vi "APC_9049_SensorCalibration.vi"() -> (0 "DAQqueues":T1={"SignalList"={"CAS"=["Pcyl1_bar", "Pcyl2_bar", "Pcyl3_bar", "Pcyl4_bar", "Pcyl5_bar", "Pcyl6_bar", "Ppre_bar", "Psyst_bar", "Pexh_bar"], "CycAvg"=["TimeStamp9049_ms", "TimeStamp9056echo_ms", "InjectionState_b", "InjEnable_b", "MainEnable_b", "MainDuration_ms", "MainSOI_CADBTDC", "SparkEnable_b", "SparkTiming_CADBTDC", "EngineSpeed_rpm", "WF_PT_012avg_bar", "WF_PT_005avg_bar", "PrechamberPeakPdiff_bar", "IMEPg1_bar", "IMEPg2_bar", "IMEPg3_bar", "IMEPg4_bar", "IMEPg5_bar", "IMEPg6_bar", "IMEPn1_bar", "IMEPn2_bar", "IMEPn3_bar", "IMEPn4_bar", "IMEPn5_bar", "IMEPn6_bar", "PMEP1_bar", "PMEP2_bar", "PMEP3_bar", "PMEP4_bar", "PMEP5_bar", "PMEP6_bar", "MaxPcyl1_bar", "MaxPcyl2_bar", "MaxPcyl3_bar", "MaxPcyl4_bar", "MaxPcyl5_bar", "MaxPcyl6_bar", "IMEPstd1_bar", "IMEPstd2_bar", "IMEPstd3_bar", "IMEPstd4_bar", "IMEPstd5_bar", "IMEPstd6_bar", "MAPO1_bar", "MAPO2_bar", "MAPO3_bar", "MAPO4_bar", "MAPO5_bar", "MAPO6_bar", "RI1", "RI2", "RI3", "RI4", "RI5", "RI6", "maxQ1_J", "maxQ2_J", "maxQ3_J", "maxQ4_J", "maxQ5_J", "maxQ6_J", "CA03_1_CADATDC", "CA03_2_CADATDC", "CA03_3_CADATDC", "CA03_4_CADATDC", "CA03_5_CADATDC", "CA03_6_CADATDC", "CA10_1_CADATDC", "CA10_2_CADATDC", "CA10_3_CADATDC", "CA10_4_CADATDC", "CA10_5_CADATDC", "CA10_6_CADATDC", "CA50_1_CADATDC", "CA50_2_CADATDC", "CA50_3_CADATDC", "CA50_4_CADATDC", "CA50_5_CADATDC", "CA50_6_CADATDC", "CA90_1_CADATDC", "CA90_2_CADATDC", "CA90_3_CADATDC", "CA90_4_CADATDC", "CA90_5_CADATDC", "CA90_6_CADATDC", "CA97_1_CADATDC", "CA97_2_CADATDC", "CA97_3_CADATDC", "CA97_4_CADATDC", "CA97_5_CADATDC", "CA97_6_CADATDC", "CA10CA90_1_CAD", "CA10CA90_2_CAD", "CA10CA90_3_CAD", "CA10CA90_4_CAD", "CA10CA90_5_CAD", "CA10CA90_6_CAD", "maxdpdcad1_barCAD", "maxdpdcad2_barCAD", "maxdpdcad3_barCAD", "maxdpdcad4_barCAD", "maxdpdcad5_barCAD", "maxdpdcad6_barCAD", "kappa_comp1_r", "kappa_comp2_r", "kappa_comp3_r", "kappa_comp4_r", "kappa_comp5_r", "kappa_comp6_r", "kappa_exp1_r", "kappa_exp2_r", "kappa_exp3_r", "kappa_exp4_r", "kappa_exp5_r", "kappa_exp6_r", "CylPresWarnings_u64", "CylPresErrors_u64", "TimeStamp9056_ms", "SystemState_i8", "WF_PT_001_bar", "WF_OA_001_O2_perc", "WF_OA_001_O2corr_perc", "WF_OA_001_Lambda_r", "WF_OA_002_O2_perc", "WF_OA_002_Lambda_r", "WF_OA_002_NOx_ppm", "EO_PT_001_bar", "TORQUE_Nm", "NI9205_9_V", "NI9205_10_V", "NI9205_11_V", "NI9205_12_V", "NI9205_13_V", "NI9205_14_V", "NI9205_15_V", "NG_FT_001_kgs", "NG_PT_001_bar", "NGDI_PT_001_bar", "O2_FC_001_kgs", "NG_FC_001_kgs", "NGDI_FT_001_kgs", "WF_PT_004_bar", "O2_PT_001_bar", "AR_PT_001_bar", "AR_FT_001_kgs", "WF_PT_016_bar", "WF_PT_014_bar", "SW_FT_001_kgs", "SW_FT_002_kgs", "SW_FT_003_kgs", "SW_FT_004_kgs", "WF_TT_001_degC", "O2_TT_001_degC", "AR_TT_001_degC", "NG_TT_001_degC", "NGDI_TT_001_degC", "WF_TT_002 _degC", "WF_TT_003_degC", "WF_TT_004_degC", "WF_TT_007_degC", "PC_TT_001_degC", "PC_TT_002_degC", "PC_TT_003_degC", "PC_TT_004_degC", "PC_TT_005_degC", "PC_TT_006_degC", "EC_TT_001_degC", "EC_TT_002_degC", "SW_TT_001_degC", "SW_TT_002_degC", "SW_TT_003_degC", "SW_TT_004_degC", "SW_TT_005_degC", "SW_TT_006_degC", "SW_TT_007_degC", "SW_TT_008_degC", "SW_TT_009_degC", "EO_TT_001_degC", "EO_TT_002_degC", "NI9214b_13_degC", "NI9214b_14_degC", "NI9214b_15_degC", "NI9214b_16_degC", "NI9264_AO0_V", "NI9264_AO1_V", "NI9264_AO2_V", "NI9264_AO3_V", "NI9264_AO4_V", "NI9264_AO5_V", "NI9264_AO6_V", "NI9264_AO7_V", "NI9264_AO8_V", "NI9264_AO9_V", "NI9264_AO10_V", "NI9264_AO11_V", "NI9264_AO12_V", "NI9264_AO13_V", "NI9264_AO14_V", "NI9264_AO15_V", "O2_FC_001_REF_mA", "AR_PC_002_REF_mA", "NG_FC_001_REF_mA", "EC_FC_001_mA", "SW_FC_004_REF_mA", "SW_FC_009_mA", "DYNO_REF_mA", "NI9266_AO7_mA", "NG_FV_001_b", "O2_PV_004_b", "AR_PV_004_b", "WF_FC_001_b", "WF_FC_002_b", "WF_FC_003_b", "NI9375_AO6_b", "NI9375_AO7_b", "NI9375_AO8_b", "NI9375_AO9_b", "NI9375_AO10_b", "NI9375_AO11_b", "NI9375_AO12_b", "NI9375_AO13_b", "NI9375_AO14_b", "NI9375_AO15_b", "NI9375_AI0_b", "NI9375_AI1_b", "NI9375_AI2_b", "NI9375_AI3_b", "NI9375_AI4_b", "NI9375_AI5_b", "NI9375_AI6_b", "NI9375_AI7_b", "NI9375_AI8_b", "NI9375_AI9_b", "NI9375_AI10_b", "NI9375_AI11_b", "NI9375_AI12_b", "NI9375_AI13_b", "NI9375_AI14_b", "NI9375_AI15_b", "AIC103_CO2_ConcTarget_ack", "AT103_CO2Conc", "PV103_PressTarget_kPa_ack", "PT103_Pressure_kPa", "PV103_VlvPosTarget_pc_ack", "PV103_VlvPos_pc_fb", "AIC201_CO2_ConcTarget_ack", "AT201_CO2Conc", "FV301_FlowTarget_kgh_ack", "FT301_Flow_kgh", "FV301_VlvPosTarget_pc_ack", "FV301_VlvPos_pc_fb", "PV300_PressTarget_kPa_ack", "PT300_Pressure_kPa", "PV300_VlvPosTarget_pc_ack", "PV300_VlvPos_pc_fb", "C101_CompSpeed_rpm", "PT104_Pressure_kPa", "PT106_Pressure_kPa", "PLC_Manual_Control", "MTR_State", "MTR_HeartBeat", "PV103_Ctrl_Mode_act", "FV301_Ctrl_Mode_act", "PV300_Ctrl_Mode_act", "MTR_Diagnostic_Status"]}, "Queues"={"CAS"=refnum, "CycAvg"=refnum}, "scaled units"=["bar", "bar", "bar", "bar", "bar", "bar", "bar", "bar", "bar"]}, 1 "error out":errorcluster, 2 "scaled dAQmx task":refnum<k21>)   [LabVIEW 2020]
doc: "This example demonstrates the procedure required to apply different NI-DAQmx Custom Scales to each virtual channel in a task. A DAQmx Task Property Node (Functions >> NI Measurements >> DAQmx - Data Acquisition >> DAQmx Advanced Task Options) is used to obtain the task's virtual channels. A DAQmx Channel Property Node (Functions >> NI Measurements >> DAQmx - Data Acquisition) is then used to set the custom scale for each virtual channel in the task.\n\nThe \"DAQmx Create Scale\" VI creates a custom scale for each channel in the channel list. *Note, make sure your Minimum and Maximum channel parameters are consistent with the range the scale will create."
uses:
  controls/APC_DAQqueues.ctl
  <vilib>/DAQmx/create/channels.llb/DAQmx Create Channel (AI-Voltage-Basic).vi
  <vilib>/DAQmx/create/scale.llb/DAQmx Create Scale (Linear).vi
  <vilib>/DAQmx/configure/timing.llb/DAQmx Timing (Sample Clock).vi
  <vilib>/DAQmx/configure/trigger.llb/DAQmx Start Trigger (Digital Edge).vi
  <resource>/objmgr/daqmx.rc
panel:
  out "CRIO9049signals":string[](array[string])=["TimeStamp9049_ms", "TimeStamp9056echo_ms", "InjectionState_b", "InjEnable_b", "MainEnable_b", "MainDuration_ms", "MainSOI_CADBTDC", "SparkEnable_b", "SparkTiming_CADBTDC", "EngineSpeed_rpm", "WF-PT-012avg_bar", "WF-PT-005avg_bar", "PrechamberPeakPdiff_bar", "IMEPg1_bar", "IMEPg2_bar", "IMEPg3_bar", "IMEPg4_bar", "IMEPg5_bar", "IMEPg6_bar", "IMEPn1_bar", "IMEPn2_bar", "IMEPn3_bar", "IMEPn4_bar", "IMEPn5_bar", "IMEPn6_bar", "PMEP1_bar", "PMEP2_bar", "PMEP3_bar", "PMEP4_bar", "PMEP5_bar", "PMEP6_bar", "MaxPcyl1_bar", "MaxPcyl2_bar", "MaxPcyl3_bar", "MaxPcyl4_bar", "MaxPcyl5_bar", "MaxPcyl6_bar", "IMEPstd1_bar", "IMEPstd2_bar", "IMEPstd3_bar", "IMEPstd4_bar", "IMEPstd5_bar", "IMEPstd6_bar", "MAPO1_bar", "MAPO2_bar", "MAPO3_bar", "MAPO4_bar", "MAPO5_bar", "MAPO6_bar", "RI1", "RI2", "RI3", "RI4", "RI5", "RI6", "maxQ1_J", "maxQ2_J", "maxQ3_J", "maxQ4_J", "maxQ5_J", "maxQ6_J", "CA03_1_CADATDC", "CA03_2_CADATDC", "CA03_3_CADATDC", "CA03_4_CADATDC", "CA03_5_CADATDC", "CA03_6_CADATDC", "CA10_1_CADATDC", "CA10_2_CADATDC", "CA10_3_CADATDC", "CA10_4_CADATDC", "CA10_5_CADATDC", "CA10_6_CADATDC", "CA50_1_CADATDC", "CA50_2_CADATDC", "CA50_3_CADATDC", "CA50_4_CADATDC", "CA50_5_CADATDC", "CA50_6_CADATDC", "CA90_1_CADATDC", "CA90_2_CADATDC", "CA90_3_CADATDC", "CA90_4_CADATDC", "CA90_5_CADATDC", "CA90_6_CADATDC", "CA97_1_CADATDC", "CA97_2_CADATDC", "CA97_3_CADATDC", "CA97_4_CADATDC", "CA97_5_CADATDC", "CA97_6_CADATDC", "CA10CA90_1_CAD", "CA10CA90_2_CAD", "CA10CA90_3_CAD", "CA10CA90_4_CAD", "CA10CA90_5_CAD", "CA10CA90_6_CAD", "maxdpdcad1_barCAD", "maxdpdcad2_barCAD", "maxdpdcad3_barCAD", "maxdpdcad4_barCAD", "maxdpdcad5_barCAD", "maxdpdcad6_barCAD", "kappa_comp1_r", "kappa_comp2_r", "kappa_comp3_r", "kappa_comp4_r", "kappa_comp5_r", "kappa_comp6_r", "kappa_exp1_r", "kappa_exp2_r", "kappa_exp3_r", "kappa_exp4_r", "kappa_exp5_r", "kappa_exp6_r", "CylPresWarnings_u64", "CylPresErrors_u64"]
  out "CRIO9056signals":string[](array[string])=["TimeStamp9056_ms", "SystemState_i8", "WF-PT-001_bar", "WF-OA-001-O2_perc", "WF-OA-001-O2corr_perc", "WF-OA-001-Lambda_r", "WF-OA-002-O2_perc", "WF-OA-002-Lambda_r", "WF-OA-002-NOx_ppm", "EO-PT-001_bar", "TORQUE_Nm", "NI9205_9_V", "NI9205_10_V", "NI9205_11_V", "NI9205_12_V", "NI9205_13_V", "NI9205_14_V", "NI9205_15_V", "NG-FT-001_kgs", "NG-PT-001_bar", "NGDI-PT-001_bar", "O2-FC-001_kgs", "NG-FC-001_kgs", "NGDI-FT-001_kgs", "WF-PT-004_bar", "O2-PT-001_bar", "AR-PT-001_bar", "AR-FT-001_kgs", "WF-PT-016_bar", "WF-PT-014_bar", "SW-FT-001_kgs", "SW-FT-002_kgs", "SW-FT-003_kgs", "SW-FT-004_kgs", "WF-TT-001_degC", "O2-TT-001_degC", "AR-TT-001_degC", "NG-TT-001_degC", "NGDI-TT-001_degC", "WF-TT-002 _degC", "WF-TT-003_degC", "WF-TT-004_degC", "WF-TT-007_degC", "PC-TT-001_degC", "PC-TT-002_degC", "PC-TT-003_degC", "PC-TT-004_degC", "PC-TT-005_degC", "PC-TT-006_degC", "EC-TT-001_degC", "EC-TT-002_degC", "SW-TT-001_degC", "SW-TT-002_degC", "SW-TT-003_degC", "SW-TT-004_degC", "SW-TT-005_degC", "SW-TT-006_degC", "SW-TT-007_degC", "SW-TT-008_degC", "SW-TT-009_degC", "EO-TT-001_degC", "EO-TT-002_degC", "NI9214b_13_degC", "NI9214b_14_degC", "NI9214b_15_degC", "NI9214b_16_degC", "NI9264_AO0_V", "NI9264_AO1_V", "NI9264_AO2_V", "NI9264_AO3_V", "NI9264_AO4_V", "NI9264_AO5_V", "NI9264_AO6_V", "NI9264_AO7_V", "NI9264_AO8_V", "NI9264_AO9_V", "NI9264_AO10_V", "NI9264_AO11_V", "NI9264_AO12_V", "NI9264_AO13_V", "NI9264_AO14_V", "NI9264_AO15_V", "O2-FC-001-REF_mA", "AR-PC-002-REF_mA", "NG-FC-001-REF_mA", "EC-FC-001_mA", "SW-FC-004-REF_mA", "SW-FC-009_mA", "DYNO-REF_mA", "NI9266_AO7_mA", "NG-FV-001_b", "O2-PV-004_b", "AR-PV-004_b", "WF-FC-001_b", "WF-FC-002_b", "WF-FC-003_b", "NI9375_AO6_b", "NI9375_AO7_b", "NI9375_AO8_b", "NI9375_AO9_b", "NI9375_AO10_b", "NI9375_AO11_b", "NI9375_AO12_b", "NI9375_AO13_b", "NI9375_AO14_b", "NI9375_AO15_b", "NI9375_AI0_b", "NI9375_AI1_b", "NI9375_AI2_b", "NI9375_AI3_b", "NI9375_AI4_b", "NI9375_AI5_b", "NI9375_AI6_b", "NI9375_AI7_b", "NI9375_AI8_b", "NI9375_AI9_b", "NI9375_AI10_b", "NI9375_AI11_b", "NI9375_AI12_b", "NI9375_AI13_b", "NI9375_AI14_b", "NI9375_AI15_b", "AIC103_CO2_ConcTarget_ack", "AT103_CO2Conc", "PV103_PressTarget_kPa_ack", "PT103_Pressure_kPa", "PV103_VlvPosTarget_pc_ack", "PV103_VlvPos_pc_fb", "AIC201_CO2_ConcTarget_ack", "AT201_CO2Conc", "FV301_FlowTarget_kgh_ack", "FT301_Flow_kgh", "FV301_VlvPosTarget_pc_ack", "FV301_VlvPos_pc_fb", "PV300_PressTarget_kPa_ack", "PT300_Pressure_kPa", "PV300_VlvPosTarget_pc_ack", "PV300_VlvPos_pc_fb", "C101_CompSpeed_rpm", "PT104_Pressure_kPa", "PT106_Pressure_kPa", "PLC_Manual_Control", "MTR_State", "MTR_HeartBeat", "PV103_Ctrl_Mode_act", "FV301_Ctrl_Mode_act", "PV300_Ctrl_Mode_act", "MTR_Diagnostic_Status"]
  out "CycAvgSignalList":string[](array[string])=["TimeStamp9049_ms", "TimeStamp9056echo_ms", "InjectionState_b", "InjEnable_b", "MainEnable_b", "MainDuration_ms", "MainSOI_CADBTDC", "SparkEnable_b", "SparkTiming_CADBTDC", "EngineSpeed_rpm", "WF_PT_012avg_bar", "WF_PT_005avg_bar", "PrechamberPeakPdiff_bar", "IMEPg1_bar", "IMEPg2_bar", "IMEPg3_bar", "IMEPg4_bar", "IMEPg5_bar", "IMEPg6_bar", "IMEPn1_bar", "IMEPn2_bar", "IMEPn3_bar", "IMEPn4_bar", "IMEPn5_bar", "IMEPn6_bar", "PMEP1_bar", "PMEP2_bar", "PMEP3_bar", "PMEP4_bar", "PMEP5_bar", "PMEP6_bar", "MaxPcyl1_bar", "MaxPcyl2_bar", "MaxPcyl3_bar", "MaxPcyl4_bar", "MaxPcyl5_bar", "MaxPcyl6_bar", "IMEPstd1_bar", "IMEPstd2_bar", "IMEPstd3_bar", "IMEPstd4_bar", "IMEPstd5_bar", "IMEPstd6_bar", "MAPO1_bar", "MAPO2_bar", "MAPO3_bar", "MAPO4_bar", "MAPO5_bar", "MAPO6_bar", "RI1", "RI2", "RI3", "RI4", "RI5", "RI6", "maxQ1_J", "maxQ2_J", "maxQ3_J", "maxQ4_J", "maxQ5_J", "maxQ6_J", "CA03_1_CADATDC", "CA03_2_CADATDC", "CA03_3_CADATDC", "CA03_4_CADATDC", "CA03_5_CADATDC", "CA03_6_CADATDC", "CA10_1_CADATDC", "CA10_2_CADATDC", "CA10_3_CADATDC", "CA10_4_CADATDC", "CA10_5_CADATDC", "CA10_6_CADATDC", "CA50_1_CADATDC", "CA50_2_CADATDC", "CA50_3_CADATDC", "CA50_4_CADATDC", "CA50_5_CADATDC", "CA50_6_CADATDC", "CA90_1_CADATDC", "CA90_2_CADATDC", "CA90_3_CADATDC", "CA90_4_CADATDC", "CA90_5_CADATDC", "CA90_6_CADATDC", "CA97_1_CADATDC", "CA97_2_CADATDC", "CA97_3_CADATDC", "CA97_4_CADATDC", "CA97_5_CADATDC", "CA97_6_CADATDC", "CA10CA90_1_CAD", "CA10CA90_2_CAD", "CA10CA90_3_CAD", "CA10CA90_4_CAD", "CA10CA90_5_CAD", "CA10CA90_6_CAD", "maxdpdcad1_barCAD", "maxdpdcad2_barCAD", "maxdpdcad3_barCAD", "maxdpdcad4_barCAD", "maxdpdcad5_barCAD", "maxdpdcad6_barCAD", "kappa_comp1_r", "kappa_comp2_r", "kappa_comp3_r", "kappa_comp4_r", "kappa_comp5_r", "kappa_comp6_r", "kappa_exp1_r", "kappa_exp2_r", "kappa_exp3_r", "kappa_exp4_r", "kappa_exp5_r", "kappa_exp6_r", "CylPresWarnings_u64", "CylPresErrors_u64", "TimeStamp9056_ms", "SystemState_i8", "WF_PT_001_bar", "WF_OA_001_O2_perc", "WF_OA_001_O2corr_perc", "WF_OA_001_Lambda_r", "WF_OA_002_O2_perc", "WF_OA_002_Lambda_r", "WF_OA_002_NOx_ppm", "EO_PT_001_bar", "TORQUE_Nm", "NI9205_9_V", "NI9205_10_V", "NI9205_11_V", "NI9205_12_V", "NI9205_13_V", "NI9205_14_V", "NI9205_15_V", "NG_FT_001_kgs", "NG_PT_001_bar", "NGDI_PT_001_bar", "O2_FC_001_kgs", "NG_FC_001_kgs", "NGDI_FT_001_kgs", "WF_PT_004_bar", "O2_PT_001_bar", "AR_PT_001_bar", "AR_FT_001_kgs", "WF_PT_016_bar", "WF_PT_014_bar", "SW_FT_001_kgs", "SW_FT_002_kgs", "SW_FT_003_kgs", "SW_FT_004_kgs", "WF_TT_001_degC", "O2_TT_001_degC", "AR_TT_001_degC", "NG_TT_001_degC", "NGDI_TT_001_degC", "WF_TT_002 _degC", "WF_TT_003_degC", "WF_TT_004_degC", "WF_TT_007_degC", "PC_TT_001_degC", "PC_TT_002_degC", "PC_TT_003_degC", "PC_TT_004_degC", "PC_TT_005_degC", "PC_TT_006_degC", "EC_TT_001_degC", "EC_TT_002_degC", "SW_TT_001_degC", "SW_TT_002_degC", "SW_TT_003_degC", "SW_TT_004_degC", "SW_TT_005_degC", "SW_TT_006_degC", "SW_TT_007_degC", "SW_TT_008_degC", "SW_TT_009_degC", "EO_TT_001_degC", "EO_TT_002_degC", "NI9214b_13_degC", "NI9214b_14_degC", "NI9214b_15_degC", "NI9214b_16_degC", "NI9264_AO0_V", "NI9264_AO1_V", "NI9264_AO2_V", "NI9264_AO3_V", "NI9264_AO4_V", "NI9264_AO5_V", "NI9264_AO6_V", "NI9264_AO7_V", "NI9264_AO8_V", "NI9264_AO9_V", "NI9264_AO10_V", "NI9264_AO11_V", "NI9264_AO12_V", "NI9264_AO13_V", "NI9264_AO14_V", "NI9264_AO15_V", "O2_FC_001_REF_mA", "AR_PC_002_REF_mA", "NG_FC_001_REF_mA", "EC_FC_001_mA", "SW_FC_004_REF_mA", "SW_FC_009_mA", "DYNO_REF_mA", "NI9266_AO7_mA", "NG_FV_001_b", "O2_PV_004_b", "AR_PV_004_b", "WF_FC_001_b", "WF_FC_002_b", "WF_FC_003_b", "NI9375_AO6_b", "NI9375_AO7_b", "NI9375_AO8_b", "NI9375_AO9_b", "NI9375_AO10_b", "NI9375_AO11_b", "NI9375_AO12_b", "NI9375_AO13_b", "NI9375_AO14_b", "NI9375_AO15_b", "NI9375_AI0_b", "NI9375_AI1_b", "NI9375_AI2_b", "NI9375_AI3_b", "NI9375_AI4_b", "NI9375_AI5_b", "NI9375_AI6_b", "NI9375_AI7_b", "NI9375_AI8_b", "NI9375_AI9_b", "NI9375_AI10_b", "NI9375_AI11_b", "NI9375_AI12_b", "NI9375_AI13_b", "NI9375_AI14_b", "NI9375_AI15_b", "AIC103_CO2_ConcTarget_ack", "AT103_CO2Conc", "PV103_PressTarget_kPa_ack", "PT103_Pressure_kPa", "PV103_VlvPosTarget_pc_ack", "PV103_VlvPos_pc_fb", "AIC201_CO2_ConcTarget_ack", "AT201_CO2Conc", "FV301_FlowTarget_kgh_ack", "FT301_Flow_kgh", "FV301_VlvPosTarget_pc_ack", "FV301_VlvPos_pc_fb", "PV300_PressTarget_kPa_ack", "PT300_Pressure_kPa", "PV300_VlvPosTarget_pc_ack", "PV300_VlvPos_pc_fb", "C101_CompSpeed_rpm", "PT104_Pressure_kPa", "PT106_Pressure_kPa", "PLC_Manual_Control", "MTR_State", "MTR_HeartBeat", "PV103_Ctrl_Mode_act", "FV301_Ctrl_Mode_act", "PV300_Ctrl_Mode_act", "MTR_Diagnostic_Status"]
  out "Min V":dbl[](array[numeric])=[-10.0, -10.0, -10.0, -10.0, -10.0, -10.0, -10.0, -10.0, -10.0]
  out "Max V":dbl[](array[numeric])=[10.0, 10.0, 10.0, 10.0, 10.0, 10.0, 10.0, 10.0, 10.0]
  out "channels name":string[](array[string])=["Pcyl1", "Pcyl2", "Pcyl3", "Pcyl4", "Pcyl5", "Pcyl6", "Ppre", "Psyst", "Pexh"]
  out "scaled units":string[](array[string])=["bar", "bar", "bar", "bar", "bar", "bar", "bar", "bar", "bar"]
  out "Y-Intercept":dbl[](array[numeric])=[0.0, 5.0, 10.0, 15.0, 0.0, 0.0, 0.0, 0.0, 0.0] format="%.2g"
  out "Slope":dbl[](array[numeric])=[1.0, 1.0, 1.0, 100.0, 1.0, 1.0, 1.0, 1.0, 1.0] format="%.2g"
  in  "Physical Channels":tag="Mod1/ai0:3, Mod2/ai0:3, Mod8/ai0"
  # "Scale Parameters"
  # "Channel Parameters"
  # "Note: maximum and minimum values are in voltage and are only used for selecting the ADC range (if the card has several available). They DO not limit the measured value."
  # "Varriables in files"
  # "List of variables recorded in the cycle averaged files and included in the data raster created by the C9049. Over that, CRIO9056 must be (manually) updated, as you will need to update the 9049 list there"
  # "List Avg signal headers. \n0) C9049 timespatmp\n1) Control settings\n2) Averaged values from analog signals and other cycle synchronous\n3) CRIO9056 signals (you will need to retrieve this from the CRIO9056)\n3) Signals retrieved from CRIO9056"
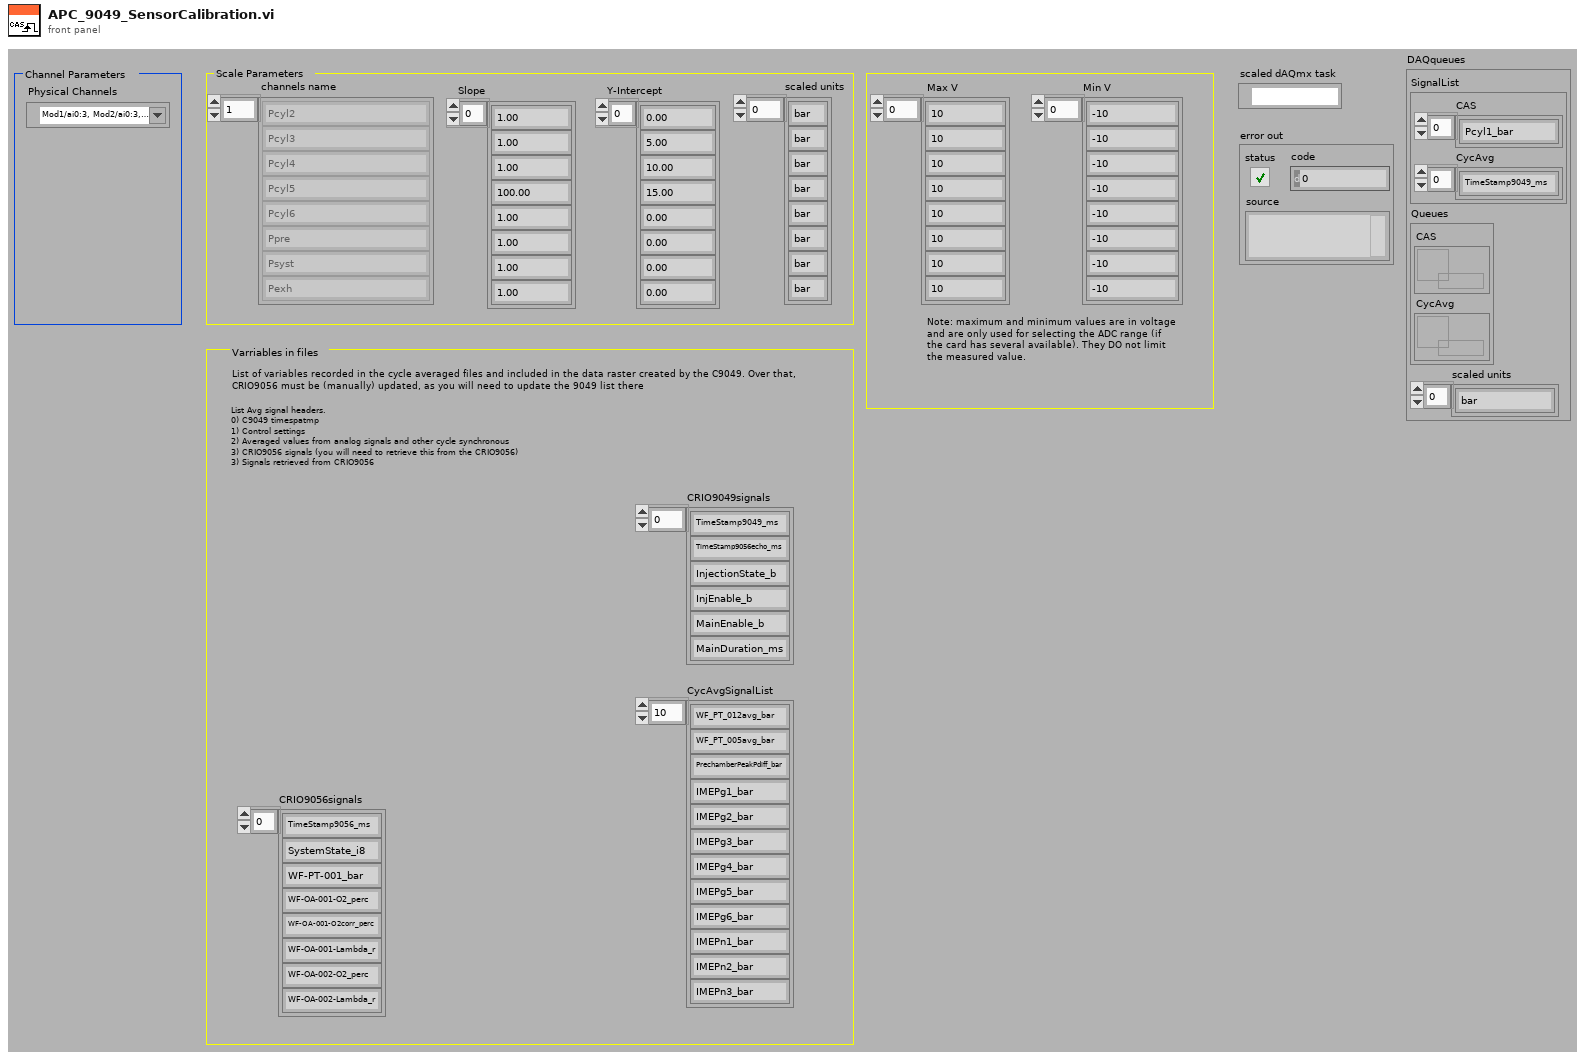
[diagram p1: front panel]
types:
  T1 = typedef "APC_DAQqueues.ctl" = cluster{"SignalList":cluster{"CAS":string[], "CycAvg":string[]}, "Queues":cluster{"CAS":refnum<queue>, "CycAvg":refnum<queue>}, "scaled units":string[]}
  T2 = cluster{"CAS":refnum<queue>, "CycAvg":refnum<queue>}
  T3 = cluster{"SignalList":cluster{"CAS":string[], "CycAvg":string[]}, "Queues":cluster{"CAS":refnum<queue>, "CycAvg":refnum<queue>}, "scaled units out":string[]}
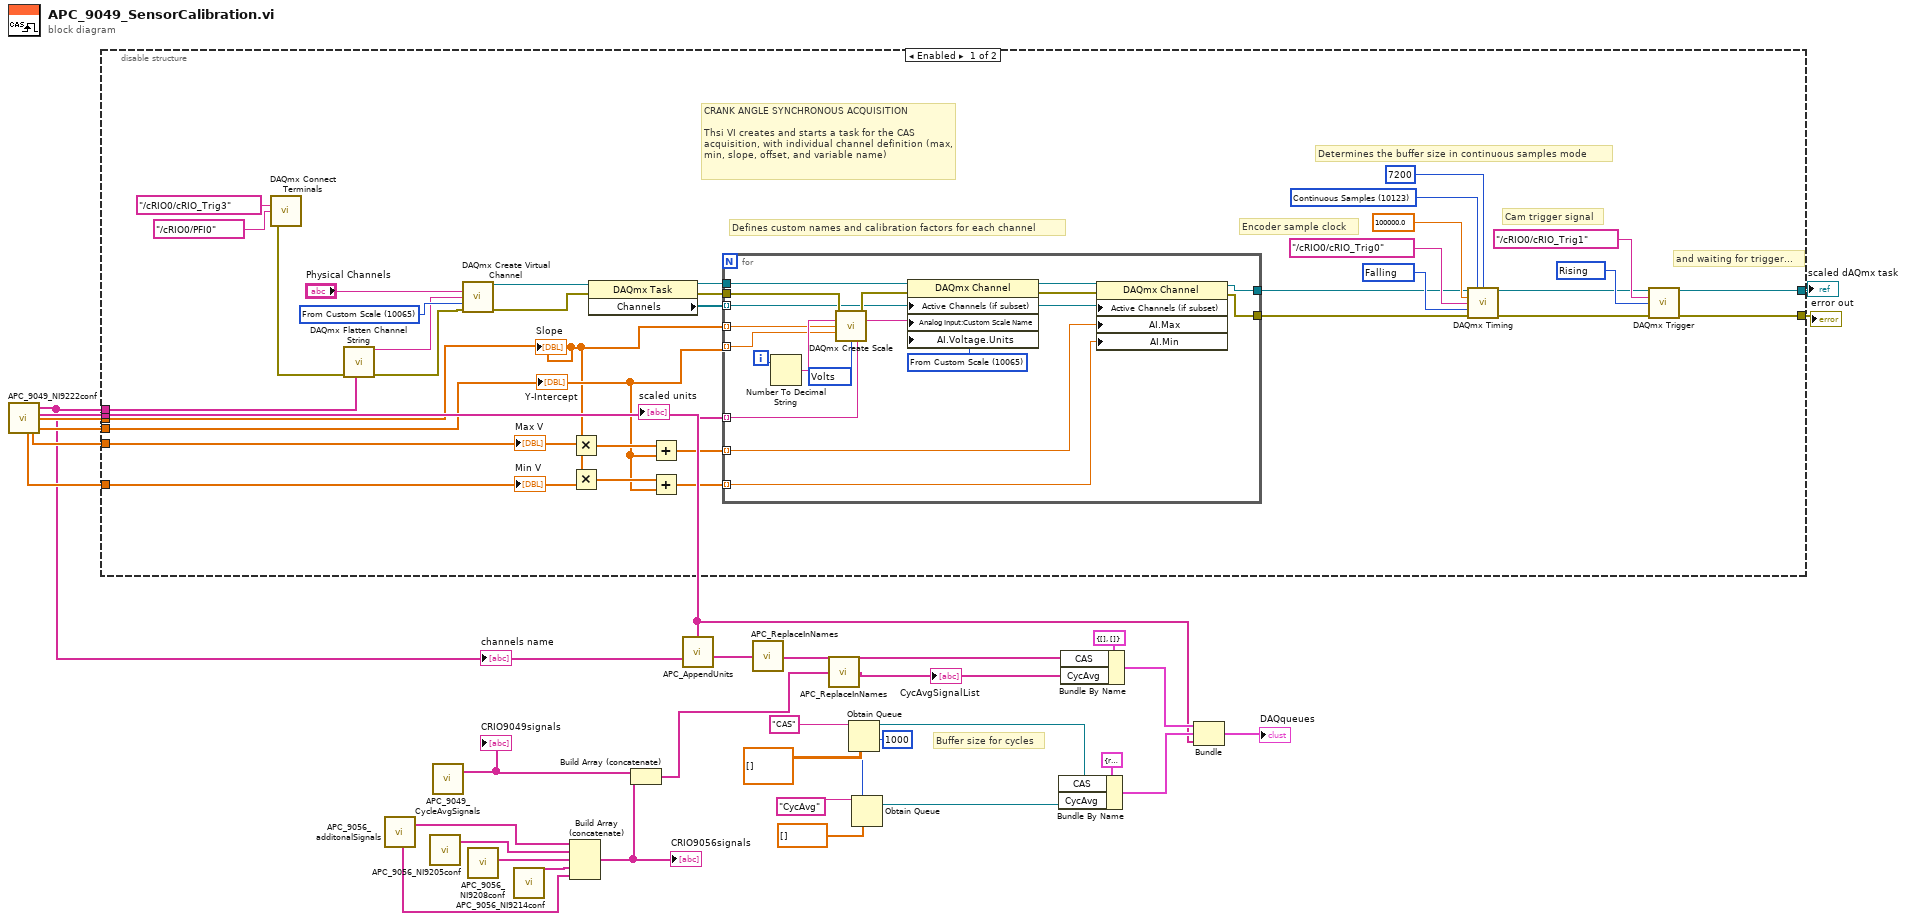
[diagram p0: block diagram]
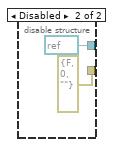
[diagram p2: hidden frame]
diagram:
  w19 = 1000 ("max queue size (-1, unlimited)")
  # "Buffer size for cycles"
  n1 = call "APC_9049_NI9222conf.vi"() -> ("Min V out"=w11:dbl[], "Max V out"=w12:dbl[], "scaled units out"=w6:string[], "Y-Intercept out"=w10:dbl[], "Slope out"=w9:dbl[], "channels name out"=w5:string[])
  "channels name" <- w5
  n2 = disable-structure shown="Enabled" {
    disable-tunnel: [w48 refnum<k21> refnum ("task out")] -> w21
    disable-tunnel: [w47 errorcluster {"status"=FALSE, "code"=0, "source"=""} ("error out")] -> w20
    disable-tunnel: w12 -> [w37 _]
    disable-tunnel: w11 -> [w36 _]
    disable-tunnel: w10 -> [w35 _]
    disable-tunnel: w9 -> [w34 _]
    disable-tunnel: w6 -> [w33 _]
    disable-tunnel: w5 -> [w32 _]
    frame Enabled {
      w54 = 10280 items=["Rising"=10280, "Falling"=10171] ("edge")
      w53 = 10123 items=["Finite Samples"=10178, "Continuous Samples"=10123, "Hardware Timed Single Point"=12522] ("sample mode")
      w50 = 10171 items=["Rising"=10280, "Falling"=10171] ("active edge")
      w60 = 10065 items=["Volts"=10348, "From Custom Scale"=10065] ("units")
      # "and waiting for trigger..."
      # "Defines custom names and calibration factors for each channel"
      # "CRANK ANGLE SYNCHRONOUS ACQUISITION\n\nThsi VI creates and starts a task for the CAS acquisition, with individual channel definition (max, min, slope, offset, and variable name)"
      # "Determines the buffer size in continuous samples mode"
      # "Encoder sample clock"
      # "Cam trigger signal"
      n3 = call <vilib>:"DAQmx Connect Terminals.vi"("source terminal"=tag "/cRIO0/cRIO_Trig3", "destination terminal"=tag "/cRIO0/PFI0") -> ("error out"=w42:errorcluster)  [unwired: 13 in]
      n4 = call <vilib>:"DAQmx Flatten Channel String.vi"("names in"=w32, "error in"=w42) -> ("names out"=w59:string, "error out"=w58:errorcluster)  [unwired: 12 in]
      n5 = call-poly <vilib>:"DAQmx Create Virtual Channel.vi"("physical channels"="Physical Channels", "name to assign"=w59, "units"=w60, "error in"=w58) -> ("task out"=w65:refnum<k21>, "error out"=w62:errorcluster)  [unwired: 10 in]
      n6 = Multiply(x=w34, y=w37) -> (x*y=w40:dbl[])
      n7 = Multiply(x=w34, y=w36) -> (x*y=w39:dbl[])
      n8 = property class="DAQmx Task"(reference=w65, error in=w62) -> (reference out=w64:refnum<k21>, error out=w61:errorcluster, "Channels"=w63:refnum<k21>[])
      n9 = Add(x=w40, y=w35) -> (x+y=w41:dbl[])
      n10 = Add(x=w39, y=w35) -> (x+y=w38:dbl[])
      n11 = for {
        tunnel: w64 -> [w73]
        tunnel: w63 -> [w71] mode=indexing
        tunnel: w61 -> [w84]
        tunnel: w35 -> [w77] mode=indexing
        tunnel: w33 -> [w81] mode=indexing
        tunnel: [w79] -> w46
        tunnel: [w78] -> w45
        tunnel: w41 -> [w74] mode=indexing
        tunnel: w34 -> [w76] mode=indexing
        tunnel: w38 -> [w75] mode=indexing
        i -> [w83]
        w69 = 10065 items=["Volts"=10348, "From Custom Scale"=10065, "From TEDS"=12516] ("AI.Voltage.Units")
        w80 = 10348 items=["Volts"=10348, "Amps"=10342, "Deg F"=10144, "Deg C"=10143, "Deg R"=10145, "Kelvins"=10325, "Strain"=10299, "Ohms"=10384, "Hz"=10373, "Seconds"=10364, "Meters"=10219, "Inches"=10379, "Degrees"=10146, "Radians"=10273, "Ticks"=10304, "g"=10186, "m/s^2"=12470, "m/s"=15959, "in/s"=15960, "Pascals"=10081, "Newtons"=15875, "Pounds"=15876, "kgf"=15877, "psi"=15879, "bar"=15880, "Nm"=15881, "oz-in"=15882, "lb-in"=15883, "lb-ft"=15884, "Volts/Volt"=15896, "mVolts/Volt"=15897, "pCoulombs"=16103, "Coulombs"=16102, "From TEDS"=12516] ("pre-scaled units")
        n12 = Number To Decimal String(number=w83) -> (decimal integer string=w82:string)  [unwired: 1 in]
        n13 = call-poly <vilib>:"DAQmx Create Scale.vi"("name"=w82, "slope"=w76, "y-intercept"=w77, "error in"=w84, "pre-scaled units"=w80, "scaled units"=w81) -> ("scale out"=w70:tag, "error out"=w72:errorcluster)  [unwired: 8 in]
        n14 = property class="DAQmx Channel"(reference=w73, error in=w72, "Active Channels (if subset)"=w71, "Analog Input:Custom Scale Name"=w70, "AI.Voltage.Units"=w69) -> (reference out=w68:refnum<k21>, error out=w67:errorcluster)
        n15 = property class="DAQmx Channel"(reference=w68, error in=w67, "Active Channels (if subset)"=w71, "AI.Max"=w74, "AI.Min"=w75) -> (reference out=w79:refnum<k21>, error out=w78:errorcluster)
      }
      n16 = call-poly <vilib>:"DAQmx Timing.vi"("task/channels in"=w46, "sample mode"=w53, "samples per channel"=7200 ("number of samples per channel"), "rate"=100000.0, "source"=tag "/cRIO0/cRIO_Trig0", "active edge"=w50, "error in"=w45) -> ("task out"=w49:refnum<k21>, "error out"=w56:errorcluster)  [unwired: 7 in]
      n17 = call-poly <vilib>:"DAQmx Trigger.vi"("task/channels in"=w49, "source"=tag "/cRIO0/cRIO_Trig1", "edge"=w54, "error in"=w56) -> ("task out"=w48:refnum<k21>, "error out"=w47:errorcluster)  [unwired: 10 in]
      "Slope" <- w34
      "Y-Intercept" <- w35
      "scaled units" <- w33
      "Max V" <- w37
      "Min V" <- w36
    }
    frame Disabled {
    }
  }
  "scaled dAQmx task" <- w21
  "error out" <- w20
  n18 = call "APC_9056_additonalSignals.vi"() -> ("AdditionalTSSignalList_post"=w13:string[], "AdditionalTSSignalList_pre"=w17:string[])  [unwired: 2 in]
  n19 = call "APC_9056_NI9205conf.vi"() -> ("channels name out"=w16:string[])  [unwired: 5 out]
  n20 = call "APC_9049_CycleAvgSignals.vi"() -> ("CRIo9049_CycleAvgSignals"=w8:string[])  [unwired: 3 in]
  "CRIO9049signals" <- w8
  n21 = call "APC_9056_NI9208conf.vi"() -> ("channels name out"=w15:string[])  [unwired: 5 out]
  n22 = call "APC_9056_NI9214conf.vi"() -> ("channels name out"=w14:string[])  [unwired: 5 in]
  n23 = Build Array (concatenate)(w17, w16, w15, w14, w13) -> (w7:string[])
  "CRIO9056signals" <- w7
  n24 = Build Array (concatenate)(w8, w7) -> (w2:string[])
  n25 = call "APC_AppendUnits.vi"("units"=w6, "names"=w5) -> ("names_units"=w4:string[])
  n26 = call "APC_ReplaceInNames.vi"("string"=w4) -> ("result string"=w3:string[])
  n27 = call "APC_ReplaceInNames.vi"("string"=w2) -> ("result string"=w1:string[])
  "CycAvgSignalList" <- w1
  n28 = Obtain Queue(max queue size (-1, unlimited)=w19, name (unnamed)="CAS", element data type=dbl[][] []) -> (queue out=w26:refnum<queue>)  [unwired: 2 in, 2 out]
  n29 = Obtain Queue(max queue size (-1, unlimited)=w19, name (unnamed)="CycAvg", element data type=dbl[] [] ("appended array")) -> (queue out=w25:refnum<queue>)  [unwired: 2 in, 2 out]
  n30 = Bundle By Name(cluster=T2 {"CAS"=refnum, "CycAvg"=refnum} ("Queues"), "CAS"=w26, "CycAvg"=w25) -> (w22:T2)
  n31 = Bundle By Name(cluster=cluster{"CAS":string[], "CycAvg":string[]} {"CAS"=[], "CycAvg"=[]} ("SignalList"), "CAS"=w3, "CycAvg"=w1) -> (w23:cluster{"CAS":string[], "CycAvg":string[]})
  n32 = Bundle("SignalList"=w23, "Queues"=w22, "scaled units out"=w6) -> (→"DAQqueues":T3)  [unwired: 1 in]
